vi "Read.vi"(8 "error in (no error)":errorcluster, 11 "Cluster in":refnum<class "Cluster.lvclass">) -> (0 "error out":errorcluster, 1 "Data Array":refnum<class "Generic Data.lvclass">[](array[class]), 2 "Name Array":string[](array[string]), 3 "Cluster out":refnum<class "Cluster.lvclass">)   [LabVIEW 2020, in "Data.lvlib" / "Cluster.lvclass"]
doc: "Read Cluster data."
uses:
  Cluster.lvclass
  Generic Data.lvclass
  Cluster.lvclass/Cluster.ctl
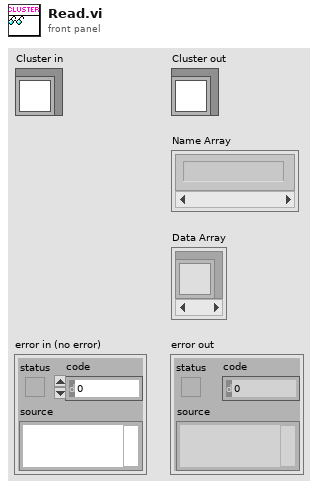
[diagram p1: front panel]
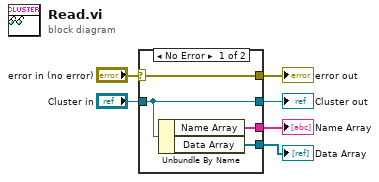
[diagram p0: block diagram]
diagram:
  n1 = case shown="No Error" "error in (no error)" {
    selector: "error in (no error)" -> [w10 w11]
    tunnel: [w10 w11] -> w5
    tunnel: [w9 w12] -> w3
    tunnel: "Cluster in" -> [w9 w12]
    tunnel: [w8 _] -> w2
    tunnel: [w7 _] -> w1
    frame No Error {
      n2 = Unbundle By Name(w9) -> ("Name Array"=w8:string[], "Data Array"=w7:refnum<class "Generic Data.lvclass">[])
    }
    frame Error {
    }
  }
  "error out" <- w5
  "Cluster out" <- w3
  "Data Array" <- w1
  "Name Array" <- w2
